vi "Do.vi"(8 "error in (no error)":errorcluster, 10 "Actor in":refnum<class "Actor.lvclass">, 11 "Verify and Check-In Msg":refnum<class "Verify and Check-In Msg.lvclass">) -> (0 "error out":errorcluster, 2 "Actor out":refnum<class "Actor.lvclass">)   [LabVIEW 2023, in "Guest Manager Model.lvlib" / "Verify and Check-In Msg.lvclass"]
doc: "This VI delivers the message to the actor by calling the appropriate method(s) on the actor."
uses:
  Verify and Check-In Msg.lvclass
  Verify and Check-In Msg.lvclass/Verify and Check-In Msg.ctl
  34700b1e-4b1b-4205-ab4b-28631ba2a4c6.vi
  Guest Manager Model/Guest Manager Model.lvclass
  Guest Manager UI/Guest Manager UI Messages/Verify and Check-in Msg/Verify and Check-in Msg.lvclass
  C:/Users/bhaghyaraj/Trainings/NI Actor Framework/SDLC/Guest Manager UI/Guest Manager UI Messages/Verify and Check-in Msg/Verify and Check-in Msg.lvclass
  C:/Program Files/National Instruments/LabVIEW 2023/vi.lib/ActorFramework/Message/Message.lvclass
  C:/Users/bhaghyaraj/Trainings/NI Actor Framework/SDLC/Guest Manager Model/Guest Manager Model Messages/Verify and Check-In Msg/Verify and Check-In Msg.lvclass
  <vilib>/ActorFramework/Actor/Actor.lvclass
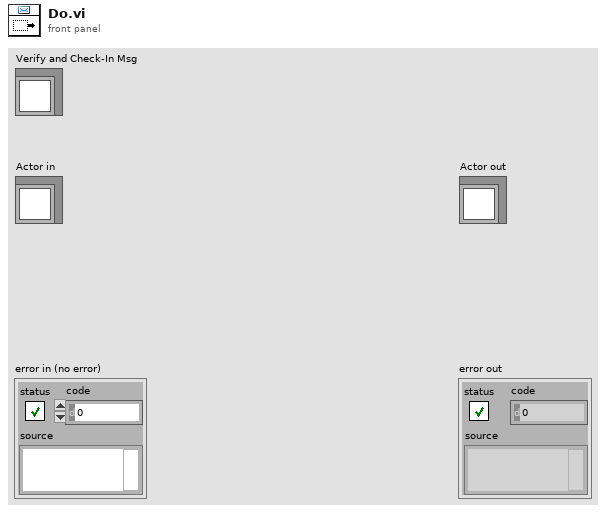
[diagram p1: front panel]
types:
  T1 = cluster{"Children":u32, "Adults":u32, "Primary Guest Name":string, "Guest Contact Number":string, "Room No":string}
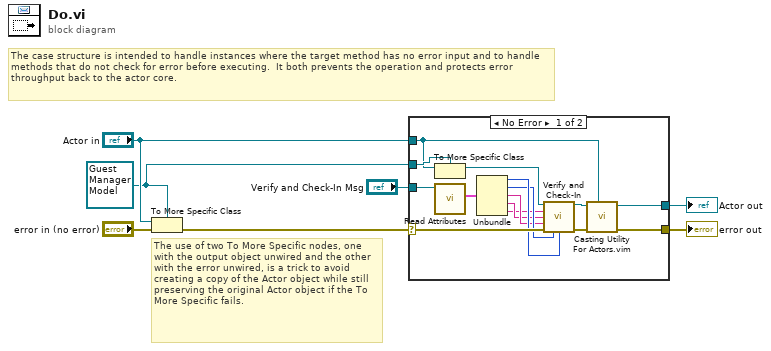
[diagram p0: block diagram]
diagram:
  w2 = refnum<class "Guest Manager Model.lvclass"> refnum ("Actor in")
  # "The use of two To More Specific nodes, one with the output object unwired and the other with the error unwired, is a trick to avoid creating a copy of the Actor object while still preserving the original Actor object if the To More Specific fails."
  # "The case structure is intended to handle instances where the target method has no error input and to handle methods that do not check for error before executing.  It both prevents the operation and protects error throughput back to the actor core."
  n1 = To More Specific Class(target class=w2, reference="Actor in", error in="error in (no error)") -> (error out=w6:errorcluster)  [unwired: 1 out]
  n2 = case shown="No Error" w6 {
    selector: w6 -> [w22 w24]
    tunnel: [w14 w24] -> w5
    tunnel: [w13 w23] -> w4
    tunnel: "Actor in" -> [w17 w23]
    tunnel: w2 -> [w18 _]
    tunnel: "Verify and Check-In Msg" -> [w19 _]
    frame No Error {
      n3 = To More Specific Class(target class=w18, reference=w17) -> (specific class reference=w21:refnum<class "Guest Manager Model.lvclass">)  [unwired: 1 in, 1 out]
      n4 = call "Read Attributes.vi"("Verify and Check-in Msg"=w19) -> ("Payload"=w20:T1)  [unwired: 10 in]
      n5 = Unbundle(w20) -> ("Children"=w12:u32, "Adults"=w11:u32, "Primary Guest Name"=w10:string, "Guest Contact Number"=w9:string, "Room No"=w8:string)
      n6 = call "Verify and Check-In.vi"("Guest Manager Model in"=w21, "Room No"=w8, "Guest Contact Number"=w9, "Primary Guest Name"=w10, "error in (no error)"=w22, "Adults"=w11, "Children"=w12) -> ("Guest Manager Model out"=w16:refnum<class "Guest Manager Model.lvclass">, "error out"=w15:errorcluster)  [unwired: 7 in]
      n7 = call "Casting Utility For Actors.vim"("type"=w17, "error in (no error)"=w15, "Actor in"=w16) -> ("error out"=w14:errorcluster, "Actor out"=w13:refnum<class "Actor.lvclass">)  [unwired: 7 in]
    }
    frame Error {
      # "If type check fails, pass the original object out again."
    }
  }
  "error out" <- w5
  "Actor out" <- w4
